vi "setListBoxColumnWidths_dev.vi"(0 "error in (no error)":errorcluster, 1 "table data":string[][](array[string]), 2 "MCListbox Refnum":refnum<vi>) -> ()   [LabVIEW 2020]
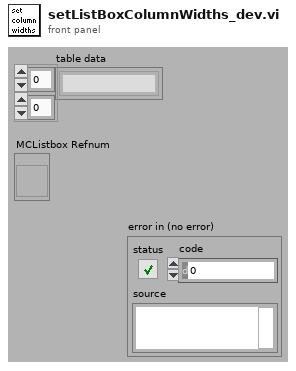
[diagram p1: front panel]
types:
  T1 = cluster{"Font Name:":string, "Size":i16, "Strikeout?":bool, "Italic?":bool, "Underline?":bool, "Outline?":bool, "Shadow?":bool, "Bold?":bool}
  T2 = enum16{"User-specified Font", "Application Font", "System Font", "Dialog Font"}
  T3 = cluster{"left":i16, "top":i16, "right":i16, "bottom":i16}
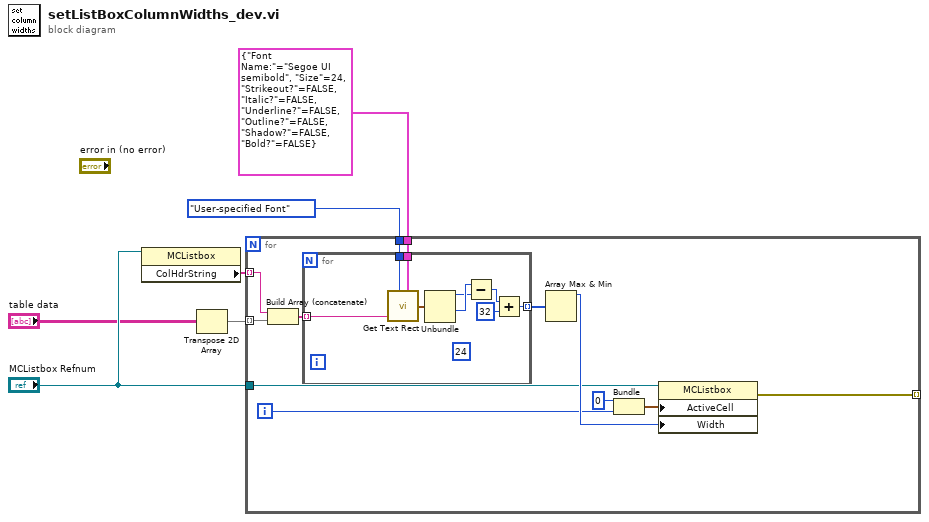
[diagram p0: block diagram]
diagram:
  n1 = property on="Property Node" class="MCListbox"(reference="MCListbox Refnum") -> ("ColHdrString"=w5:string[])  [unwired: 1 in, 2 out]
  n2 = Transpose 2D Array(2D array="table data") -> (transposed array=w3:string[][])
  n3 = for {
    tunnel: w3 -> [w11] mode=indexing
    tunnel: "MCListbox Refnum" -> [w13]
    tunnel: w5 -> [w12] mode=indexing
    tunnel: [w9] -> _ mode=indexing
    tunnel: T2."User-specified Font" ("desired font(Application)") -> [w8]
    tunnel: T1 {"Font Name:"="Segoe UI semibold", "Size"=24, "Strikeout?"=FALSE, "Italic?"=FALSE, "Underline?"=FALSE, "Outline?"=FALSE, "Shadow?"=FALSE, "Bold?"=FALSE} ("[user-specified font]") -> [w7]
    i -> [w14]
    n4 = Build Array (concatenate)(w12, w11) -> (w10:string[])
    n5 = for {
      tunnel: [w22] -> w17 mode=indexing
      tunnel: w10 -> [w21] mode=indexing
      tunnel: w8 -> [w20]
      tunnel: w7 -> [w19]
      (unwired) i16 24 ("y")
      n6 = call <vilib>:"Get Text Rect.vi"("desired font(Application)"=w20, "text"=w21, "[user-specified font]"=w19) -> ("rect"=w27:T3)  [unwired: 6 in]
      n7 = Unbundle(w27) -> ("left"=w25:i16, "right"=w26:i16)  [unwired: 2 out]
      n8 = Subtract(x=w26, y=w25) -> (x-y=w24:i16)
      n9 = Add(x=w24, y=i16 32) -> (x+y=w22:i16)
    }
    n10 = Array Max & Min(array=w17) -> (max value=w16:i16)  [unwired: 3 out]
    n11 = Bundle(0, w14) -> (w18:cluster{i32, i32})  [unwired: 1 in]
    n12 = property on="Property Node" class="MCListbox"(reference=w13, "ActiveCell"=w18, "Width"=w16) -> (error out=w9:errorcluster)  [unwired: 1 in, 1 out]
  }
